vi "Configure Harmonics.vi"(0 "VISA resource name":refnum<visa-resource-name>, 1 "PLL Source (0: U1)":i32(ring) items=["U1", "I1", "U2", "I2", "U3", "I3"], 7 "Maximum Order (50)":i32=50 min=1 max=50, 9 "Distortion Factor (0: 1/Total)":i32(ring) items=["1/Total", "1/Fundamental"], 11 "error in (no error)":errorcluster) -> (4 "VISA resource name out":refnum<visa-resource-name>, 15 "error out":errorcluster)   [LabVIEW 2016, in "Yokogawa WT300 Series.lvlib"]
doc: "Configures the harmonics features.\n\n<b>Note:</b>\nThis setting valid on models with the harmonic measurement (/G5) option."
uses:
  Yokogawa WT300 Series.lvlib
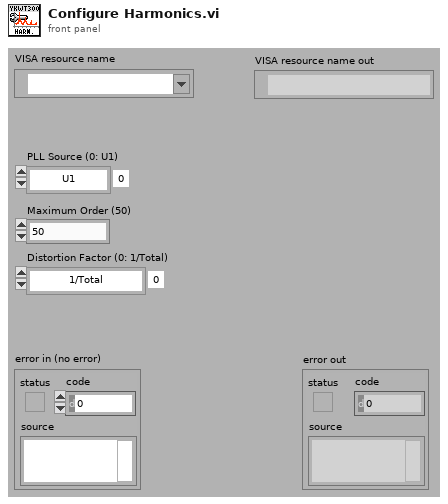
[diagram p1: front panel]
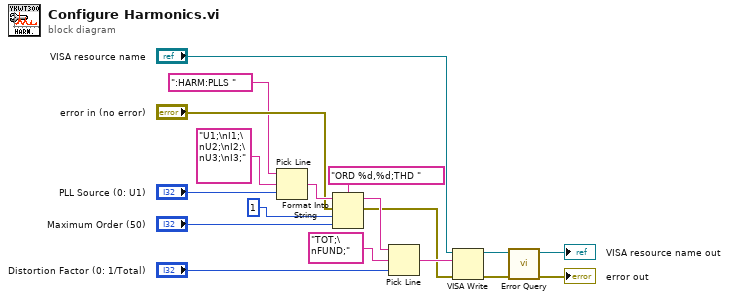
[diagram p0: block diagram]
diagram:
  n1 = Pick Line ("ライン選択")(string ("")=":HARM:PLLS " ("Œ`Ž®•¶Žš—ñ"), multi-line string="U1;\nI1;\nU2;\nI2;\nU3;\nI3;" ("¡s¶ñ"), line index="PLL Source (0: U1)") -> (output string=w9:string)
  n2 = Format Into String(format string="ORD %d,%d;THD " ("Œ`Ž®•¶Žš—ñ"), initial string=w9, error in="error in (no error)", 1, "Maximum Order (50)") -> (resulting string=w5:string, error out=w4:errorcluster)
  n3 = Pick Line ("ライン選択")(string ("")=w5, multi-line string="TOT;\nFUND;" ("¡s¶ñ"), line index="Distortion Factor (0: 1/Total)") -> (output string=w12:string)
  n4 = VISA Write ("VISA書き込み")(VISA resource name="VISA resource name", write buffer=w12, error in (no error)=w4) -> (VISA resource name out=w18:refnum<visa-resource-name>, error out=w17:errorcluster)  [unwired: 1 out]
  n5 = call "Error Query.vi"("error in (no error)"=w17, "VISA resource name"=w18) -> ("error out"=→"error out":errorcluster, "VISA resource name out"=→"VISA resource name out":refnum<visa-resource-name>)  [unwired: 6 in, 2 out]
